vi "RX.vi"(8 "error in (no error)":errorcluster, 9 "RX":bool=TRUE, 10 "Data":u8[](array[numeric]), 11 "Vision Receiver in":refnum<class "Vision Receiver.lvclass">) -> (0 "error out":errorcluster, 3 "Vision Receiver out":refnum<class "Vision Receiver.lvclass">)   [LabVIEW 2022 SP3, in "Vision Receiver.lvlib" / "Vision Receiver.lvclass"]
uses:
  Vision Receiver.lvclass
  Vision Receiver.lvclass/Vision Receiver.ctl
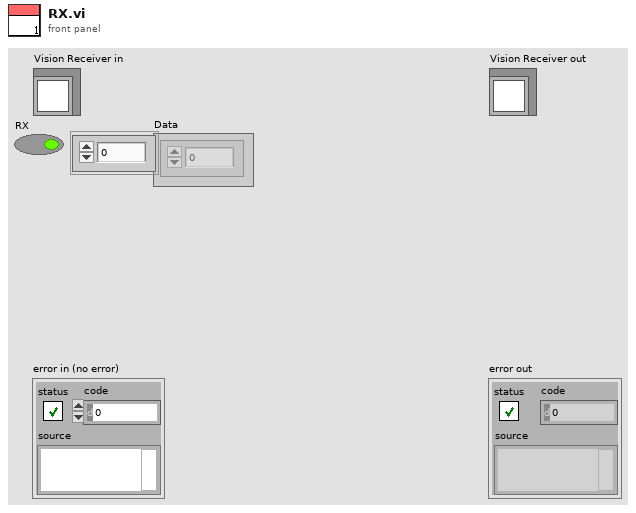
[diagram p1: front panel]
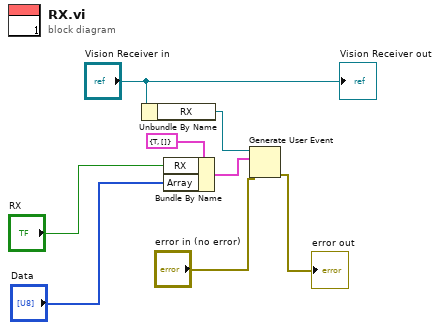
[diagram p0: block diagram]
diagram:
  n1 = Unbundle By Name("Vision Receiver in") -> ("RX"=w6:refnum<user-event>)
  n2 = Bundle By Name(cluster=cluster{"RX":bool, "Array":u8[]} {"RX"=TRUE, "Array"=[]} ("input cluster"), "RX"="RX", "Array"="Data") -> (w8:cluster{"RX":bool, "Array":u8[]})
  n3 = Generate User Event(user event=w6, event data cluster=w8, error in="error in (no error)") -> (error out=→"error out":errorcluster)  [unwired: 1 in, 1 out]
  "Vision Receiver out" <- "Vision Receiver in"
